vi "Entry.vi"(8 "error in (no error)":errorcluster, 11 "New State":refnum<class "Command Processor Actor.lvclass">) -> (0 "error out":errorcluster, 3 "State out":refnum<class "Command Processor Actor.lvclass">)   [LabVIEW 2014, in "Robot Actor Framework.lvlib" / "Command Processor Actor.lvlib" / "Command Processor Actor.lvclass"]
doc: "This is an abstract method. Override this method to define the behavior when you enter the state."
uses:
  Command Processor Actor.lvclass
  Command Processor Actor.lvclass/Command Processor Actor.ctl
  <vilib>/ni/Actors/State Actor/State Actor/State Actor.lvclass
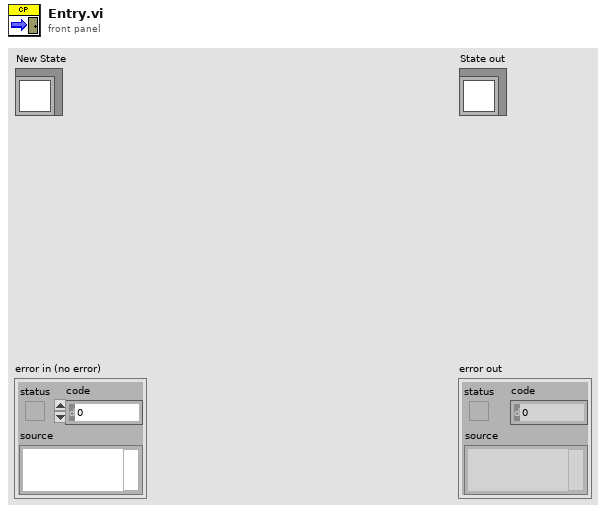
[diagram p1: front panel]
types:
  T1 = enum16{"Critical", "Error", "Warning", "Informational", "Debug"}
  T2 = typedef "Robot Actor Framework.lvlib/Command Processor Actor.lvlib/Command Processor Actor.lvclass/Command Processor States.ctl" = enum16{"Unknown", "No Command", "Running Command", "Starting Command", "Stopping Command", "Finishing Command"}
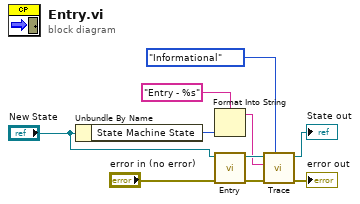
[diagram p0: block diagram]
diagram:
  n1 = Unbundle By Name("New State") -> ("State Machine State"=w2:T2)
  n2 = Format Into String(format string="Entry - %s", w2) -> (resulting string=w1:string)  [unwired: 2 in, 1 out]
  n3 = call-parent "Entry.vi"("error in (no error)"="error in (no error)", "New State"="New State") -> ("error out"=w6:errorcluster, "State out"=w9:refnum<class "Command Processor Actor.lvclass">)  [unwired: 8 in]
  n4 = call-dynamic "Trace.vi"("Trace Level"=T1."Informational", "error in (no error)"=w6, "Command Processor Action"=w1, "Command Processor Actor in"=w9) -> ("error out"=→"error out":errorcluster, "Command Processor Actor out"=→"State out":refnum<class "Command Processor Actor.lvclass">)  [unwired: 6 in]
